vi "Child_3 - SET - Triggered Events & Data.vi"(8 "error in (no error)":errorcluster, 9 "Data":string, 10 "Events":T1, 11 "Child_2_Class in":refnum<class "Child_3_Class.lvclass">) -> (0 "error out":errorcluster, 3 "Child_2_Class out":refnum<class "Child_3_Class.lvclass">)   [LabVIEW 2023, in "Actor_Child_3.lvlib" / "Child_3_Class.lvclass"]
uses:
  Child_3_Class.lvclass
  Usr Ev/Child_2 - Ctrl - Enum - Events (Temp).ctl
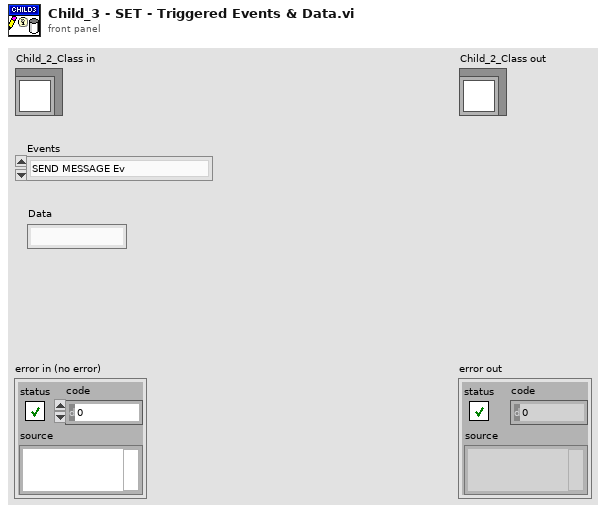
[diagram p1: front panel]
types:
  T1 = typedef "Actor_Child_3.lvlib/Child_3_Class.lvclass/Child_2 - Ctrl - Enum - Events (Temp).ctl" = enum16{"SEND MESSAGE Ev", "STOP_ACTOR Ev", "INIT_ACTOR Ev", "START Ev", "STOP Ev", "GET Ev", "SET Ev", "ERROR_HANDLER Ev", "RESET Ev", "T2 Ev", "T3 Ev", "T4 Ev"}
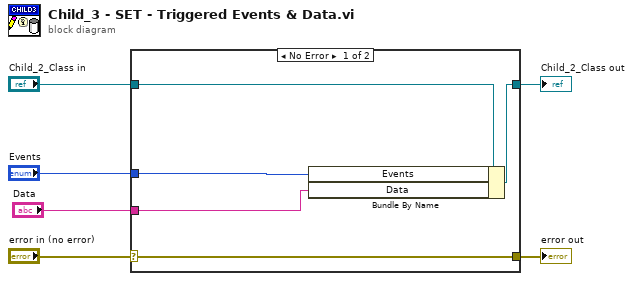
[diagram p0: block diagram]
diagram:
  n1 = case shown="No Error" "error in (no error)" {
    selector: "error in (no error)" -> [w11 w12]
    tunnel: [w11 w12] -> w5
    tunnel: [w9 w13] -> w3
    tunnel: "Child_2_Class in" -> [w10 w13]
    tunnel: "Events" -> [w8 _]
    tunnel: "Data" -> [w7 _]
    frame No Error {
      n2 = Bundle By Name(cluster=w10, "Events"=w8, "Data"=w7) -> (w9:refnum<class "Child_3_Class.lvclass">)
    }
    frame Error {
    }
  }
  "error out" <- w5
  "Child_2_Class out" <- w3
